vi "DFD MRate Filter Design.vi"   [LabVIEW 2017, in "NI_DigFilterLicensed.lvlib"]
doc: "Creates a single-stage multirate filter. You must manually select the polymorphic instance you want to use."
uses:
  <vilib>/addons/Digital Filter Design/NI_DigFilterLicensed.lvlib
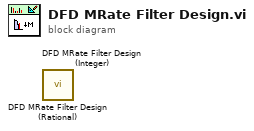
[diagram p0: block diagram]
diagram:
  n1 = call <vilib>:"DFD MRate Filter Design (Rational).vi"() -> ()  [unwired: 10 in, 2 out]
  n2 = call <vilib>:"DFD MRate Filter Design (Integer).vi"() -> ()  [unwired: 10 in, 2 out]
